vi "Create.vi"(5 "Fact In":refnum<class "Fact.lvclass">, 8 "error in (no error)":errorcluster, 10 "Path":path) -> (0 "error out":errorcluster, 3 "Fact":refnum<class "Fact.lvclass">)   [LabVIEW 2019, in "TestCase.lvlib" / "Fact.lvclass"]
uses:
  Fact.lvclass
  Fact.lvclass/Fact.ctl
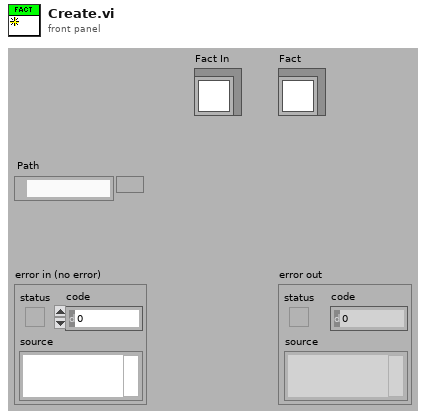
[diagram p1: front panel]
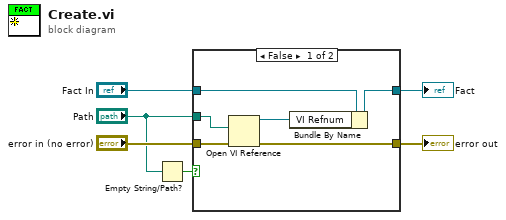
[diagram p0: block diagram]
diagram:
  n1 = Empty String/Path?(string/path="Path") -> (empty?=w1:bool)
  n2 = case shown="False" w1 {
    tunnel: "error in (no error)" -> [w12 w13]
    tunnel: "Fact In" -> [w11 w14]
    tunnel: [w10 w14] -> w4
    tunnel: [w9 w13] -> w3
    tunnel: "Path" -> [w7 _]
    frame False {
      n3 = Open VI Reference(vi path=w7, error in (no error)=w12) -> (vi reference=w8:refnum<vi>, error out=w9:errorcluster)  [unwired: 4 in]
      n4 = Bundle By Name(cluster=w11, "VI Refnum"=w8) -> (w10:refnum<class "Fact.lvclass">)
    }
    frame True {
    }
  }
  "error out" <- w3
  "Fact" <- w4
